vi "List_Box.vi"() -> ()   [LabVIEW 2017]
panel:
  out "element":i32
  out "Item Names":string[](array[string])
  out "Array":i32[](array[numeric])
  out "Listbox 2":i32[](listbox)
  in  "Listbox":i32[](listbox)
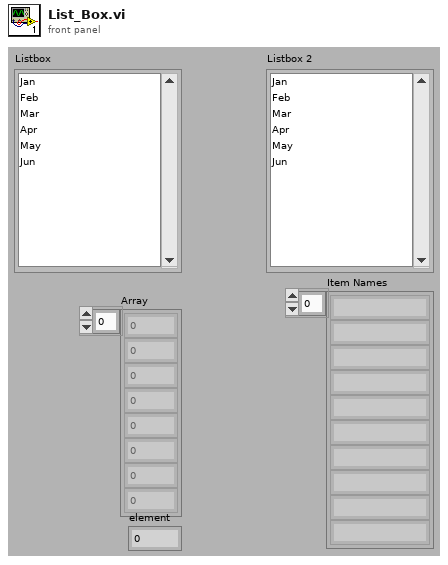
[diagram p1: front panel]
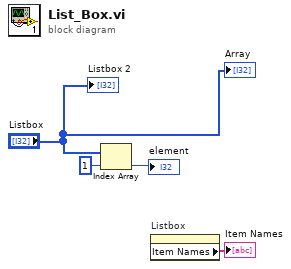
[diagram p0: block diagram]
diagram:
  n1 = Index Array(array="Listbox", index=1) -> (element=→"element":i32)
  n2 = property on="Listbox" class="LstBox (strict)"() -> ("Item Names"=→"Item Names":string[])  [unwired: 2 in, 2 out]
  "Listbox 2" <- "Listbox"
  "Array" <- "Listbox"
